vi "Pack Volts.vi"(6 "Servo Error":dbl[][](array[numeric]), 9 "Volts LVDT & LC":dbl[][](array[numeric]), 10 "L2 Cmd  Volts":dbl[](array[numeric]), 11 "L1 Cmd  Volts":dbl[](array[numeric])) -> (3 "Volts Data":dbl[][](array[numeric]))   [LabVIEW 2013]
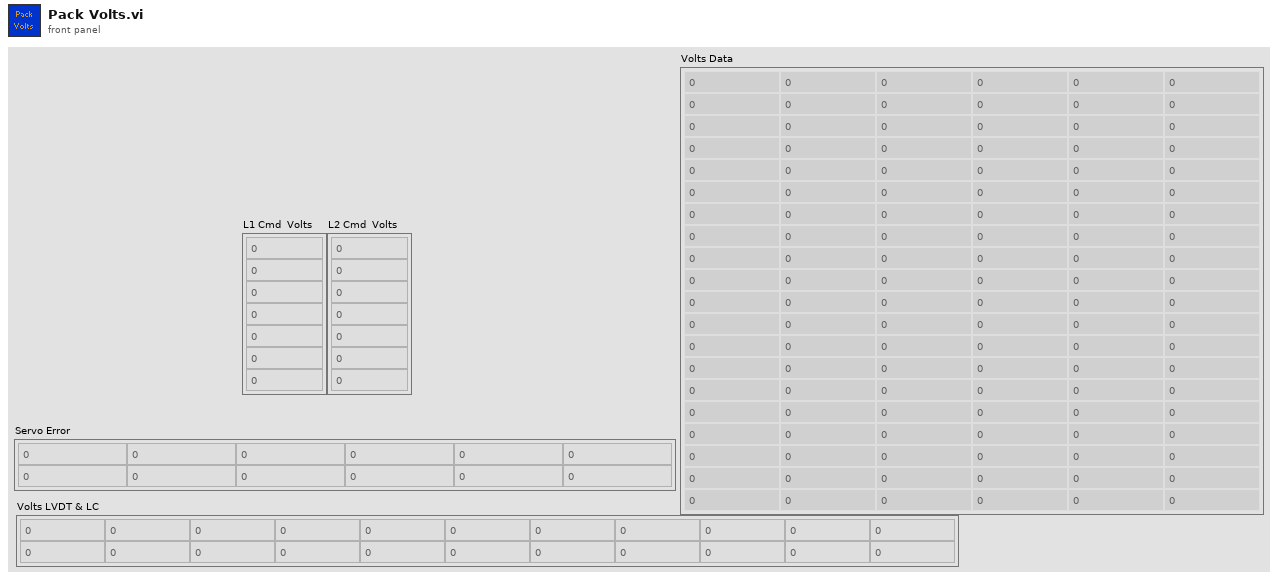
[diagram p1: front panel]
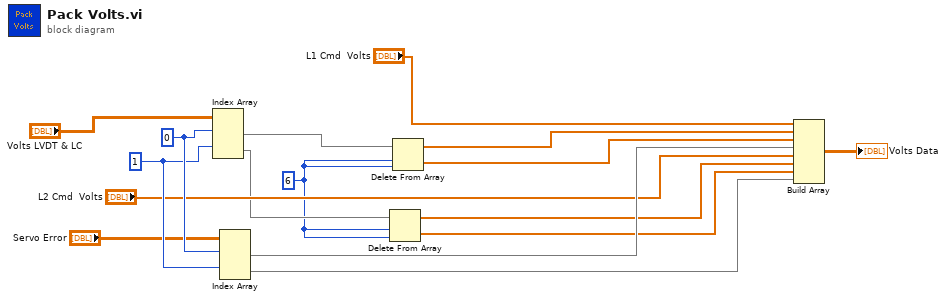
[diagram p0: block diagram]
diagram:
  w5 = 6 ("length")
  w14 = 1 ("index (row)")
  w15 = 0 ("length")
  n1 = Index Array(array="Volts LVDT & LC", index (row) #1=w15, index (row) #2=w14) -> (element #1=w12:dbl[], element #2=w6:dbl[])  [unwired: 2 in]
  n2 = Index Array(array="Servo Error", index (row) #1=w15, index (row) #2=w14) -> (element #1=w8:dbl[], element #2=w2:dbl[])  [unwired: 2 in]
  n3 = Delete From Array(array=w6, length=w5, index=w5) -> (deleted portion=w3:dbl[], array with subset deleted=w4:dbl[])
  n4 = Delete From Array(array=w12, length=w5, index=w5) -> (deleted portion=w9:dbl[], array with subset deleted=w10:dbl[])
  n5 = Build Array("L1 Cmd  Volts", w10, w9, w8, "L2 Cmd  Volts", w4, w3, w2) -> (→"Volts Data":dbl[][])
